vi "CAN Motor.vi"() -> ()   [LabVIEW 2015]
doc: "This example shows how to run a motor using CAN Jaguar. For details setting up and understanding CAN Jaguar, see the Can Jaguar Fundamentals tutorial accessable from the LabVIEW Getting Started Window.\n\n<B>Control Mode</B> Notice there are two control modes: Percent VBus and Voltage. <B>Percent VBus</B> provides the full range of the battery voltage to the motor. For example if the battery is fully charged at 13.6 volts, then half throttle would provide 6.8 volts to the motor. If the battery voltage were to lower over time to 11 volts, half throttle would only provide 5.5 volts to the motor. <B>Voltage</B> mode provides the motor with a specific voltage, as long as the battery is at or above that voltage. For example a throttle setting of 6 volts would be maintained as the battery voltage might change from 13.6 to 11 volts over time. Notice that changing the <B>Control Mode</B> will change the <B>Speed</B> range when you run the example.\n\nThis example expects a USB cable connected from your development PC to the Type B USB Jack (next to the power input) on the roboRIO.\n\nThis example requires the Driver Station to be running with Teleoperated Enabled."
uses:
  <vilib>/Rock Robotics/WPI/MotorControl/WPI_MotorControlOpenCANTalonSRX.vi
  <vilib>/Rock Robotics/WPI/CAN/TalonSRX/WPI_CANTalonSRX_APIControlMode.ctl
  <vilib>/Rock Robotics/WPI/Joystick/WPI_JoystickDeviceEnum.ctl
panel:
  out "current (A)":dbl(graph)
  out "Joystick":dbl
  in  "Device Number":u8=2
  in  "stop":bool
  # "Set these inputs before running."
  # "This can be set while running."
  # "Percent VBus"
  # "Voltage"
  # "Power\nTerminals"
  # "Motor\nTerminals"
  # "Looking at the RJ12 socket on the Jaguar, standard wire colors are shown for an inserted cable.  CAN only uses pins 3 and 4.\npin 3 (red) = CAN H\npin 4 (green) = CAN L"
  # "To roboRIO CAN terminals"
  # "Terminator plug"
  # "Black Jaguar"
  # "white\nblack\nred\ngreen\nyellow\nblue"
  # "1   2   3   4   5   6"
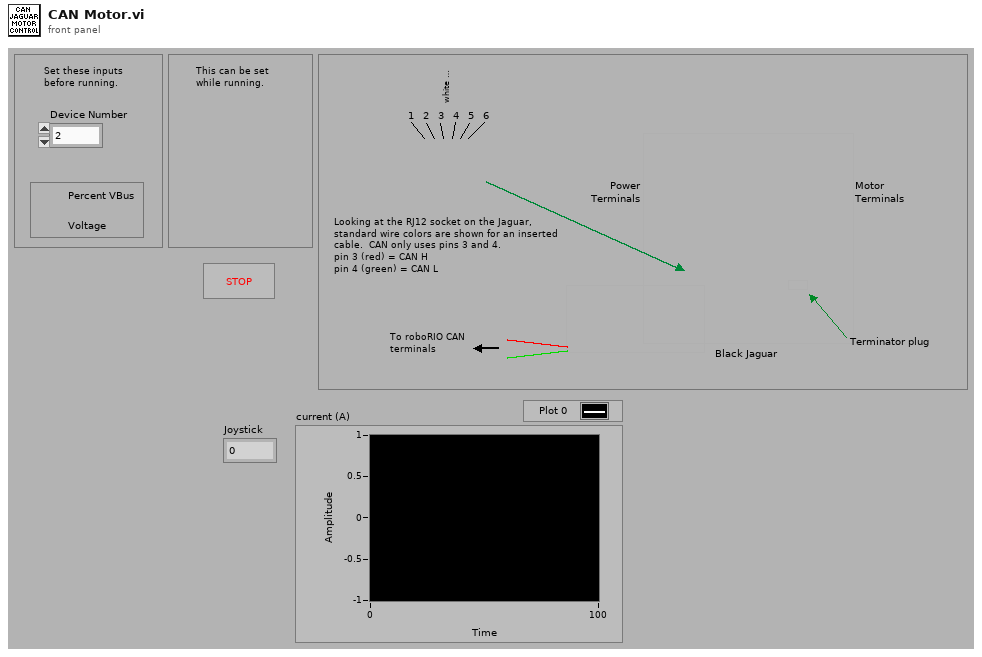
[diagram p1: front panel]
types:
  T1 = typedef "WPI_JoystickDeviceEnum.ctl" = enum16{"USB 0", "USB 1", "USB 2", "USB 3", "USB 4", "USB 5"}
  T2 = typedef "WPI_CANTalonSRX_APIControlMode.ctl" = enum8{"Percent VBus", "Speed", "Position", "Slave", "Unchanged / Invalid", "Voltage Compensation", "Current", "Motion Profile"}
  T3 = typedef "WPI_MotorControlDeviceRef.ctl" = cluster{"DeviceStatus":errorcluster, "Type":T4, "PWM":cluster{"PWM Channel":T5, "DeadBand":T6}, "CAN":cluster{"Device Number":u8, "Control Mode":T7, "Semaphore":T8, "Max Vout":dbl, "TalonSRX Control Mode":T2}, "Invert":bool}
  T4 = typedef "WPI_MotorControlType.ctl" = enum16{"PWM", "CAN", "CANTalonSRX"}
  T5 = typedef "FPGA_DIOPWMChannel.ctl" = enum8{"PWM 0", "PWM 1", "PWM 2", "PWM 3", "PWM 4", "PWM 5", "PWM 6", "PWM 7", "PWM 8", "PWM 9", "PWM MXP 0", "PWM MXP 1", "PWM MXP 2", "PWM MXP 3", "PWM MXP 4", "PWM MXP 5", "PWM MXP 6", "PWM MXP 7", "PWM MXP 8", "PWM MXP 9", "Invalid"}
  T6 = typedef "WPI_PWMDeadband.ctl" = cluster{"Name":string, "maxPositivePwm":i32, "minPositivePwm":i32, "centerPwm":i32, "maxNegativePwm":i32, "minNegativePwm":i32, "angularRange":u16}
  T7 = typedef "WPI_CANJaguar_ControlMode.ctl" = enum8{"Percent VBus", "Current", "Speed", "Position", "Voltage"}
  T8 = typedef "Semaphore RefNum" = refnum<k1>
  T9 = typedef "WPI_JoystickDevRef.ctl" = cluster{"Device":T1}
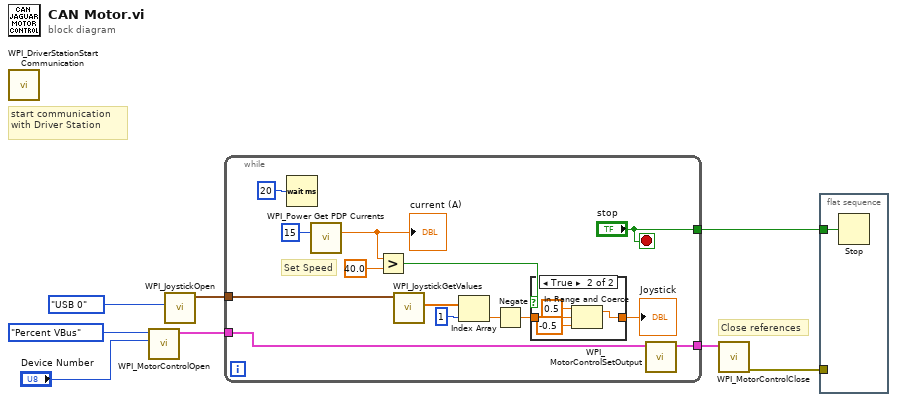
[diagram p0: block diagram]
diagram:
  # "start communication with Driver Station"
  # "Close references"
  n1 = call <vilib>:"WPI_DriverStationStart Communication.vi"() -> ()  [unwired: 2 in, 10 out]
  n2 = call-poly <vilib>:"WPI_MotorControlOpen.vi"("Device Number"="Device Number", "Control Mode"=WPI_CANTalonSRX_APIControlMode."Percent VBus") -> ("MotorControlDeviceRef"=w8:T3)  [unwired: 3 in, 6 out]
  n3 = call <vilib>:"WPI_JoystickOpen.vi"("JoystickDevice"=WPI_JoystickDeviceEnum."USB 0") -> ("JoystickDevRef"=w1:T9)  [unwired: 10 in]
  n4 = while {
    tunnel: w8 -> [w22]
    tunnel: [w21] -> w7
    tunnel: ["stop"] -> w5
    tunnel: w1 -> [w18]
    stop <- "stop" stop-if-true
    # "Set Speed"
    n5 = Wait (ms)(milliseconds to wait=u32 20) -> ()  [unwired: 1 out]
    n6 = call <vilib>:"WPI_Power Get PDP Currents.vi"("PDP Channel"=15) -> ("current (A)"=w13:dbl)  [unwired: 12 in, 2 out]
    "current (A)" <- w13
    n7 = Greater?(x=w13, y=40.0) -> (0:w10:bool)
    n8 = call <vilib>:"WPI_JoystickGetValues.vi"("JoystickDevRef"=w18) -> ("Axes"=w17:dbl[])  [unwired: 6 in, 4 out]
    n9 = Index Array(array=w17, index=1) -> (element=w15:dbl)
    n10 = Negate(x=w15) -> (-x=w11:dbl)
    n11 = case shown="True" w10 {
      tunnel: w11 -> [w23 w27]
      tunnel: [w23 w24] -> w9
      frame False {
      }
      frame True {
        n12 = In Range and Coerce(upper limit=0.5, x=w27, lower limit=-0.5) -> (coerced(x)=w24:dbl)  [unwired: 1 out]
      }
    }
    "Joystick" <- w9
    n13 = call <vilib>:"WPI_MotorControlSetOutput.vi"("MotorControlDevRef"=w22) -> ("MotorControlDevRef"=w21:T3)  [unwired: 3 in, 7 out]
  }
  n14 = call <vilib>:"WPI_MotorControlClose.vi"("MotorControlDevRef"=w7) -> ("error out"=w4:errorcluster)  [unwired: 1 in, 9 out]
  n15 = flat-sequence {
    tunnel: w5 -> [w28]
    tunnel: w4 -> [_]
    frame #0 {
      n16 = Stop(stop? (T)=w28) -> ()
    }
  }
